vi "Index_Update.vi"(8 "error in (no error)":errorcluster, 11 "StepIndexIn":u32) -> (0 "error out":errorcluster, 2 "Pause?":bool, 3 "StepIndexOut":u32)   [LabVIEW 2016, in "SeqProcessor.lvlib"]
uses:
  SeqProcessor.lvlib
  controls/StepIndex.ctl
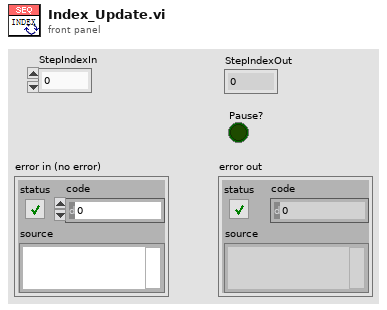
[diagram p1: front panel]
types:
  T1 = typedef "SeqProcessor.lvlib/StepIndex.ctl" = cluster{"Index1":u32, "Index2":u32}
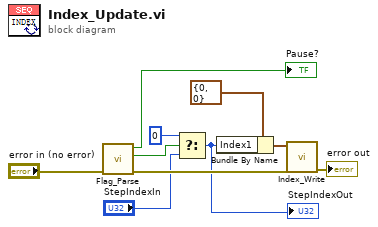
[diagram p0: block diagram]
diagram:
  n1 = call "Flag_Parse.vi"("error in (no error)"="error in (no error)") -> ("error out"=w10:errorcluster, "Stop?"=w9:bool, "Pause?"=→"Pause?":bool)  [unwired: 8 in]
  n2 = Select(t=u32 0, s=w9, f="StepIndexIn") -> (s? t:f=w4:u32)
  "StepIndexOut" <- w4
  n3 = Bundle By Name(cluster=T1 {"Index1"=0, "Index2"=0} ("Index"), "Index1"=w4) -> (w5:T1)
  n4 = call "Index_Write.vi"("error in (no error)"=w10, "Index"=w5) -> ("error out"=→"error out":errorcluster)  [unwired: 9 in]
